vi "Open Command.vi"   [LabVIEW 2020, in "SLSC.lvlib"]
doc: "Opens a reference to a command on the given resource. This allows the application to programmatically get information about the command at run time."
uses:
  <vilib>/SLSC/SLSC.lvlib
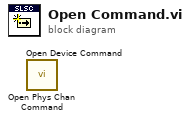
[diagram p0: block diagram]
diagram:
  n1 = call <vilib>:"Open Phys Chan Command.vi"() -> ()  [unwired: 13 in, 3 out]
  n2 = call <vilib>:"Open Device Command.vi"() -> ()  [unwired: 13 in, 3 out]
